vi "Desply Message To User Defined.vi"(8 "error in (no error)":errorcluster, 9 "Enable":bool=TRUE, 10 "Message":string="Shut Down the Program?", 11 "Show 'Cancel' Button":bool=TRUE) -> (0 "error out":errorcluster, 2 "關閉/Close":bool)   [LabVIEW 2019]
doc: "Displays a standard dialog box that contains an alert or a message for users.\n--------------------\n\nThis Express VI is configured as follows:\n\nMessage: Shut Down the Program?"
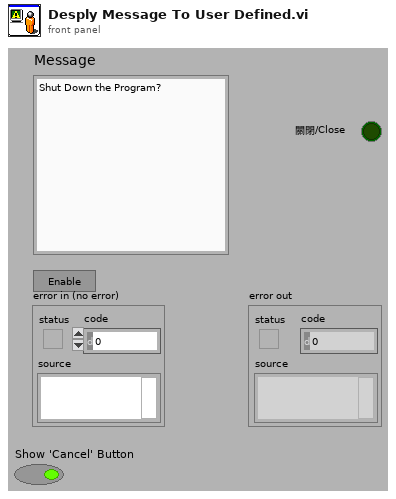
[diagram p1: front panel]
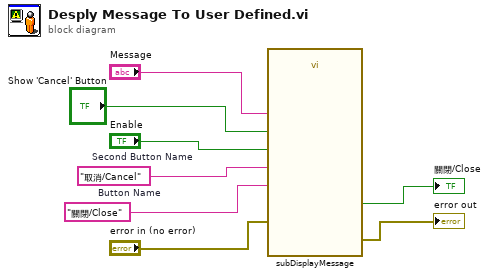
[diagram p0: block diagram]
diagram:
  w3 = "關閉/Close"  # Button Name
  w4 = "取消/Cancel"  # Second Button Name
  n1 = call <vilib>:"subDisplayMessage.vi"("Second Button Name"=w4, "Button Name"=w3, "error in (no error)"="error in (no error)", "Enable Message"="Enable", "Show 'Cancel' Button"="Show 'Cancel' Button", "Message to Display"="Message") -> ("error out"=→"error out":errorcluster, "OK?"=→"關閉/Close":bool)  [unwired: 4 in]
